vi "SysDef.Table.Set.vi"(8 "error in (no error)":errorcluster, 9 "Values":dbl[](array[numeric]), 10 "Names":string[](array[string]), 11 "nodeID":u64) -> (0 "error out":errorcluster, 3 "nodeID out":u64)   [LabVIEW 2027, in "Advanced System Definition.lvlib"]
uses:
  Advanced System Definition.lvlib
  C:/NetCore/niveristand-custom-device-development-tools/advanced-sysdef-api/Source/SysDef API/SysDef.Table.Set.vi/NationalInstruments.VeriStand.SystemDefinitionAPI
  NationalInstruments.VeriStand.SystemDefinitionAPI
  <vilib>/NI VeriStand/Custom Device API/Custom Device API.lvlib
  _Types/Dictionary Item.ctl
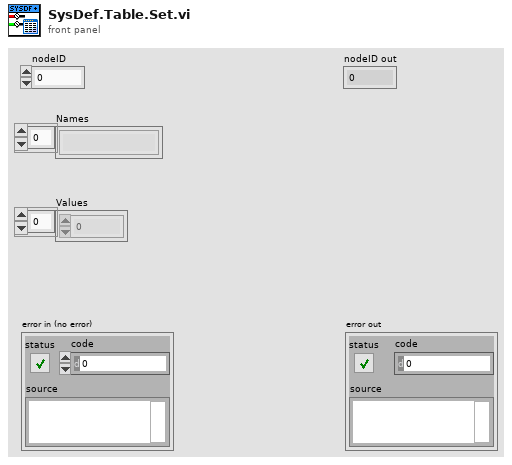
[diagram p1: front panel]
types:
  T1 = typedef "Advanced System Definition.lvlib/Dictionary Item.ctl" = cluster{"index":i32, "key":string, "value":variant}
  T2 = typedef "Custom Device API.lvlib/Custom Device Item Ref.ctl" = u64
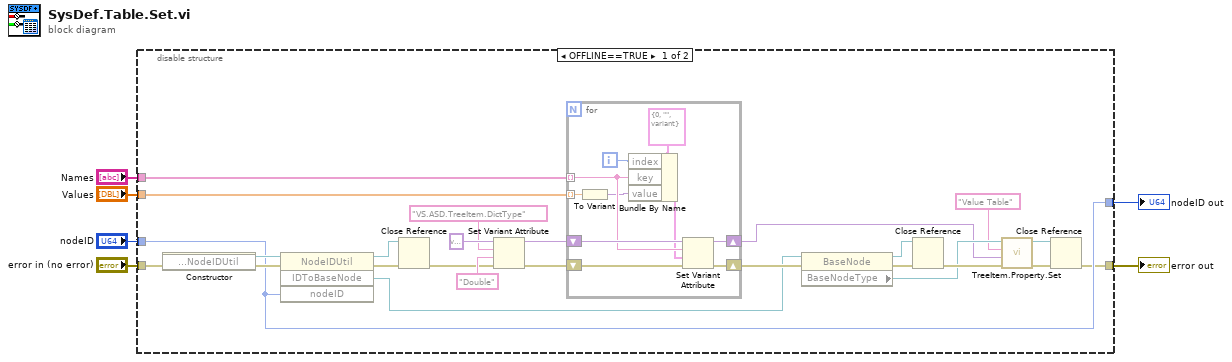
[diagram p0: block diagram]
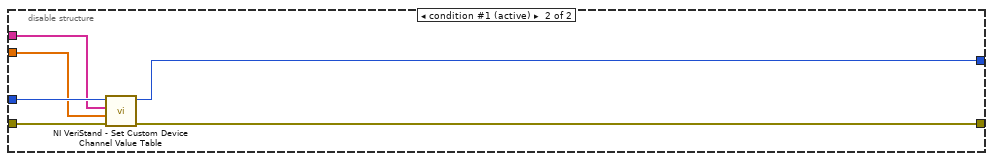
[diagram p2: hidden frame]
diagram:
  n1 = disable-structure shown="OFFLINE==TRUE" {
    disable-tunnel: "error in (no error)" -> [w27 w46]
    disable-tunnel: "nodeID" -> [w26 w47]
    disable-tunnel: [w25 w45] -> w4
    disable-tunnel: [w26 w44] -> w3
    disable-tunnel: "Names" -> [w19 w43]
    disable-tunnel: "Values" -> [w18 w42]
    frame condition #0 {
      n2 = constructor class="NodeIDUtil"(error in=w27) -> (reference out=w31:refnum<k39>, error out=w30:errorcluster)  [unwired: 2 in, 1 out]
      n3 = invoke class="NodeIDUtil" method="IDToBaseNode"(reference=w31, error in=w30, "nodeID"=w26) -> (reference out=w28:refnum<k39>, error out=w29:errorcluster, "IDToBaseNode"=w13:refnum<k39>)  [unwired: 1 in, 1 out]
      n4 = Close Reference(reference=w28, error in (no error)=w29) -> (error out=w17:errorcluster)
      n5 = Set Variant Attribute(Variant=variant, name="VS.ASD.TreeItem.DictType", value="Double" ("Type"), error in=w17) -> (Variant out=w21:variant, error out=w22:errorcluster)  [unwired: 1 out]
      n6 = for {
        tunnel: w19 -> [w38] mode=indexing
        shift-right: [w39] -> w14
        shift-left: w22 -> [w33]
        shift-right: [w40] -> w8
        shift-left: w21 -> [w41]
        tunnel: w18 -> [w34] mode=indexing
        i -> [w37]
        n7 = To Variant(anything=w34) -> (Variant=w32:variant)
        n8 = Bundle By Name(cluster=T1 {"index"=0, "key"="", "value"=variant} ("Dictionary Item"), "index"=w37, "key"=w38, "value"=w32) -> (w36:T1)
        n9 = Set Variant Attribute(Variant=w41, name=w38, value=w36, error in=w33) -> (Variant out=w40:variant, error out=w39:errorcluster)  [unwired: 1 out]
      }
      n10 = property class="BaseNode"(reference=w13, error in=w14) -> (reference out=w12:refnum<k39>, error out=w16:errorcluster, "BaseNodeType"=w11:refnum<k39>)
      n11 = Close Reference(reference=w12, error in (no error)=w16) -> (error out=w15:errorcluster)
      n12 = call "TreeItem.Property.Set.vi"("error in (no error)"=w15, "Value"=w8, "Property Name"="Value Table", "NationalInstruments.VeriStand.SystemStorage.BaseNodeType"=w11) -> ("error out"=w9:errorcluster, "NationalInstruments.VeriStand.SystemStorage.BaseNodeType"=w10:refnum<k39>)  [unwired: 5 in, 1 out]
      n13 = Close Reference(reference=w10, error in (no error)=w9) -> (error out=w25:errorcluster)
    }
    frame condition #1 (active) {
      n14 = call <vilib>:"NI VeriStand - Set Custom Device Channel Value Table.vi"("error in (no error)"=w46, "Values"=w42, "Names"=w43, "Channel Ref in"=w47) -> ("error out"=w45:errorcluster, "Channel Ref out"=w44:T2)  [unwired: 6 in]
    }
  }
  "nodeID out" <- w3
  "error out" <- w4
